vi "path steer61.vi"(11 "lane":bool) -> (2 "curve vel limit":dbl=14.843332236967187, 3 "handle":dbl=-359.09688121459806)   [LabVIEW 2015]
uses:
  G_ALL.vi
  <vilib>/Analysis/polynomials.llb/Scalar Polynomial Evaluation (DBL).vi
  <vilib>/Analysis/polynomials.llb/nth Derivative of Polynomial (DBL).vi
  G_LCM.vi
  <vilib>/Analysis/polynomials.llb/1D Polynomial Evaluation (DBL).vi
  <vilib>/Analysis/NI_AALPro.lvlib
  G_SEN.vi
  <vilib>/gmath/NI_Gmath.lvlib
panel:
  in  "speed gain":dbl=1.0 format="%#_13g"
  in  "lpf gain":dbl=0.1 format="%#_13g"
  out "Waveform Chart":dbl(graph)
  in  "index (row)":i32
  out "dist speed":dbl[](array[numeric])=[-6.280629727990325, -5.767652620171672, -5.260811269352596, -4.750405616087261, -4.247626177640517, -3.7442417201726186, -3.234236998487254, -2.733202494381619, -2.2309876435732536, -1.727969770767316, -1.2170174151123292, -0.7112755506690004, -0.2048354308747279, 0.2980698513495696, 0.8052753145152414, 1.3068201262418702, 1.8071308154794987, 2.3105942059932456, 2.816881132611934, 3.321235349091914, 3.8262467144530254, 4.328309326210711, 4.83288013729348, 5.334580351902129, 5.8405154661100145, 6.344513436357381, 6.84671687285963, 7.347037647467956, 7.85260944831298, 8.355677730085302, 8.85924459600933, 9.36378646133383, 9.871392236798886, 10.379135157785838, 10.885149114578343, 11.386372469681485, 11.889282638845971, 12.390546046536894, 12.8945305329367, 13.394897794033318, 13.897303578434707, 14.398578387722258, 14.903133677335356, 15.408547950712162, 15.909840311837332, 16.412650077140604, 16.91886527417174, 17.42043178538479, 17.928892627599016, 18.429060187867897, 18.938769393907265, 19.44497971039645, 19.95108288625684, 20.458874628420645, 20.966711680341415, 21.468694651165553, 21.97077515459592, 22.476640025076534, 22.986901398368484, 23.490789085466282, 23.998423060461953, 24.50111144191703, 25.010444092843613]
  out "Polynomial Coefficients 2":dbl[](array[numeric])
  out "R0":dbl
  out "handle 2":dbl=-359.09688121459806
  out "dist":dbl[](array[numeric])=[-6.280629727990325, -5.767652620171672, -5.260811269352596, -4.750405616087261, -4.247626177640517, -3.7442417201726186, -3.234236998487254, -2.733202494381619, -2.2309876435732536, -1.727969770767316, -1.2170174151123292, -0.7112755506690004, -0.2048354308747279, 0.2980698513495696, 0.8052753145152414, 1.3068201262418702, 1.8071308154794987, 2.3105942059932456, 2.816881132611934, 3.321235349091914, 3.8262467144530254, 4.328309326210711, 4.83288013729348, 5.334580351902129, 5.8405154661100145, 6.344513436357381, 6.84671687285963, 7.347037647467956, 7.85260944831298, 8.355677730085302, 8.85924459600933, 9.36378646133383, 9.871392236798886, 10.379135157785838, 10.885149114578343, 11.386372469681485, 11.889282638845971, 12.390546046536894, 12.8945305329367, 13.394897794033318, 13.897303578434707, 14.398578387722258, 14.903133677335356, 15.408547950712162, 15.909840311837332, 16.412650077140604, 16.91886527417174, 17.42043178538479, 17.928892627599016, 18.429060187867897, 18.938769393907265, 19.44497971039645, 19.95108288625684, 20.458874628420645, 20.966711680341415, 21.468694651165553, 21.97077515459592, 22.476640025076534, 22.986901398368484, 23.490789085466282, 23.998423060461953, 24.50111144191703, 25.010444092843613]
  in  "ap[g]":dbl=0.01 format="%#_13g"
  in  "mu":dbl=0.35 format="%#_13g"
  in  "an[g]":dbl=-0.03 format="%#_13g"
  out "Waveform Graph 2":dynamicdata(graph)=[{"t0"=timestamp(3558070004.848593 s since 1904-01-01), "dt"=1.0, "Y"=[2.6999392249698047, 1.6951051020445074, 1.0707905056587288, 0.8180527212240709, 0.9190152508675626, 1.2963877361766827, 1.970624056488019, 3.4965104940836413, 201.6, 201.6, 201.6, 201.6, 201.6, 201.6, 201.6, 201.6, 201.6, 201.6, 201.6, 201.6, 201.6, 201.6, 201.6, 201.6, 201.6, 9.532169956190149, 6.2694973959061215, 4.816384979354145, 3.8625477434998605, 3.1463412301935363, 2.568397389060611, 2.09391085834571, 1.7118919309961866, 1.427834339946269, 1.2511128718613436, 1.190295122332855, 1.2494808598163556, 1.4335700986818793, 1.7728772048959551, 2.418642872855935, 5.241778140587992, 201.6, 201.6, 201.6, 201.6, 201.6, 201.6, 201.6, 201.6, 201.6, 201.6, 201.6, 201.6, 201.6, 201.6, 201.6, 201.6, 201.6, 201.6, 201.6, 201.6, 201.6, 201.6]}, {"t0"=timestamp(3558070004.848593 s since 1904-01-01), "dt"=1.0, "Y"=[2.6999392249698047, 1.6951051020445074, 1.0707905056587288, 0.8180527212240709, 0.9190152508675626, 1.2963877361766827, 1.970624056488019, 3.4965104940836413, 20.777549661712815, 20.247536270100138, 19.694565186792815, 19.13150029565853, 18.550539773696645, 17.955042408424784, 17.333744168195455, 16.696661871332914, 16.035950098109442, 15.342378965317303, 14.611756797060403, 13.845642849689991, 13.03348797188081, 12.172479477913956, 11.240920032490967, 10.230903985827208, 9.099530123436892, 7.81122506851608, 6.2694973959061215, 4.816384979354145, 3.8625477434998605, 3.1463412301935363, 2.568397389060611, 2.09391085834571, 1.7118919309961866, 1.427834339946269, 1.2511128718613436, 1.190295122332855, 1.2494808598163556, 1.4335700986818793, 1.7728772048959551, 2.418642872855935, 5.241778140587992, 201.6, 201.6, 201.6, 201.6, 201.6, 201.6, 201.6, 201.6, 201.6, 201.6, 201.6, 201.6, 201.6, 201.6, 201.6, 201.6, 201.6, 201.6, 201.6, 201.6, 201.6, 201.6]}, {"t0"=timestamp(0 s since 1904-01-01), "dt"=1.0, "Y"=[2.6999392249698047, 1.6951051020445074, 1.0707905056587288, 0.8180527212240709, 0.9190152508675626, 1.2963877361766827, 1.970624056488019, 3.4965104940836413, 7.108855050211476, 9.429067355168725, 11.308583683012714, 12.902067626338482, 14.32116957022803, 15.603166352532973, 16.797313219711075, 16.696661871332914, 16.035950098109442, 15.342378965317303, 14.611756797060403, 13.845642849689991, 13.03348797188081, 12.172479477913956, 11.240920032490967, 10.230903985827208, 9.099530123436892, 7.81122506851608, 6.2694973959061215, 4.816384979354145, 3.8625477434998605, 3.1463412301935363, 2.568397389060611, 2.09391085834571, 1.7118919309961866, 1.427834339946269, 1.2511128718613436, 1.190295122332855, 1.2494808598163556, 1.4335700986818793, 1.7728772048959551, 2.418642872855935, 5.241778140587992, 8.106464321213798, 10.208013173205686, 11.948130714804863, 13.453538277833673, 14.81058095698709, 16.061404030280418, 17.21131827924602, 18.303446987203408, 19.317614592377343, 20.299067875936583, 21.228923087902636, 22.11953935666036, 22.978461118838254, 23.806486212234905, 24.597587927766437, 25.364173907146245, 26.113789179785613, 26.848724907341754, 27.555251257689754, 28.249167970580274, 28.919921293974994, 29.58403363562809]}]
  out "map_track for speed":dbl[][](array[numeric])=[[-0.3545450857664302, -6.2388566107065655], [-0.27704582904833586, -5.731767488012998], [-0.20533240909466363, -5.230025183339917], [-0.13399376942622507, -4.724629566643976], [-0.06871872109144915, -4.226105412976658], [-0.005201324439524461, -3.7267443688985153], [0.05648658324735591, -3.2204841411632317], [0.11292137912439827, -2.7226380925511173], [0.1614318645585973, -2.2227716212056117], [0.20611921619876952, -1.7217426590032276], [0.2514800464586248, -1.2128077861289897], [0.2966935930855752, -0.7090910317401496], [0.3370616547081277, -0.204262333528494], [0.37465481783960886, 0.29723589874642653], [0.4044573002719885, 0.803565034690598], [0.43241637259429494, 1.3043299380582118], [0.4571121863051213, 1.8040307510959646], [0.45201550718714745, 2.307468343503967], [0.3863546760099802, 2.809479406443939], [0.25417130196906557, 3.2962038986449116], [0.06111432793630125, 3.7628573931364953], [-0.19013433422201217, 4.19753080604394], [-0.49758286654376527, 4.597614676463535], [-0.8530000954510649, 4.951707459126808], [-1.2554532803579177, 5.2583045461104865], [-1.6928943683564668, 5.508622840575976], [-2.155745510638023, 5.703500011438359], [-2.634513106918592, 5.848766890858279], [-3.129308121801891, 5.952597228699951], [-3.627772088541141, 6.020504297462557], [-4.130029041586696, 6.056802252968919], [-4.634539834160694, 6.06240172093335], [-5.142102959732917, 6.055821687131267], [-5.649843095559644, 6.057503437117642], [-6.155823778443234, 6.063306282752706], [-6.656719729677723, 6.081419751160103], [-7.158588084773581, 6.113773922489787], [-7.651740703683538, 6.203582042123632], [-8.131423336348554, 6.35819424879321], [-8.583409716824091, 6.572846776944994], [-9.005194999840848, 6.845809681440183], [-9.386776083797882, 7.170882459126112], [-9.72476913428849, 7.54549791275371], [-10.011412061388244, 7.961766359884512], [-10.239416063440592, 8.40820583660063], [-10.40783468222519, 8.881970365592638], [-10.516838106738941, 9.376310409640807], [-10.590206702194822, 9.872481765496081], [-10.62912705284488, 10.379450831978916], [-10.637432741269066, 10.879549426143232], [-10.61938203200132, 11.388938910345853], [-10.592347246602534, 11.894426798329851], [-10.558291863385081, 12.399382890965526], [-10.517428444424214, 12.90552776587841], [-10.478548864380736, 13.41187433647924], [-10.440437467355913, 13.912408475588894], [-10.405933723810719, 14.413302000807835], [-10.372241554466061, 14.918043622740504], [-10.343427469450347, 15.427490791324738], [-10.315674147163909, 15.930613593740642], [-10.290940898551378, 16.43764467659748], [-10.26753174415437, 16.939787704369788], [-10.243318891221465, 17.44854450978152]]
  out "Polynomial Coefficients":dbl[](array[numeric])=[0.3514314245197786, 0.08317550338697662, -0.0038021171840465, -0.00346461088477799, -0.0012982677212205788, -0.00011561582792426496]
  out "XY Graph":cluster{"Y":dbl[], "Y":dbl[]}[](graph)=[{"Y"=[-0.3545450857664302, -0.27704582904833586, -0.20533240909466363, -0.13399376942622507, -0.06871872109144915, -0.005201324439524461, 0.05648658324735591, 0.11292137912439827, 0.1614318645585973, 0.20611921619876952, 0.2514800464586248, 0.2966935930855752, 0.3370616547081277, 0.37465481783960886, 0.4044573002719885, 0.43241637259429494, 0.4571121863051213, 0.45201550718714745, 0.3863546760099802, 0.25417130196906557, 0.06111432793630125, -0.19013433422201217, -0.49758286654376527, -0.8530000954510649, -1.2554532803579177, -1.6928943683564668], "Y"=[-6.2388566107065655, -5.731767488012998, -5.230025183339917, -4.724629566643976, -4.226105412976658, -3.7267443688985153, -3.2204841411632317, -2.7226380925511173, -2.2227716212056117, -1.7217426590032276, -1.2128077861289897, -0.7090910317401496, -0.204262333528494, 0.29723589874642653, 0.803565034690598, 1.3043299380582118, 1.8040307510959646, 2.307468343503967, 2.809479406443939, 3.2962038986449116, 3.7628573931364953, 4.19753080604394, 4.597614676463535, 4.951707459126808, 5.2583045461104865, 5.508622840575976]}, {"Y"=[-0.34824861454222367, -0.2838190821086385, -0.21088307053199773, -0.13573975147394757, -0.06474548918773154, 0.0006618412479036939, 0.06025418227747581, 0.11267247761975072, 0.16039640436065217, 0.20497730506502992, 0.2486380781866307, 0.29146844512109193, 0.33431047405158726, 0.3757168715400785, 0.41343550897313974, 0.4415691081325965, 0.4528064519658091, 0.43617827243140883, 0.3771483424612058, 0.2619623140505302, 0.07848992524601944, -0.17634937336605716, -0.5008339909423127, -0.875287479505389, -1.27737354646982, -1.6668168609056053], "Y"=[-6.2388566107065655, -5.731767488012998, -5.230025183339917, -4.724629566643976, -4.226105412976658, -3.7267443688985153, -3.2204841411632317, -2.7226380925511173, -2.2227716212056117, -1.7217426590032276, -1.2128077861289897, -0.7090910317401496, -0.204262333528494, 0.29723589874642653, 0.803565034690598, 1.3043299380582118, 1.8040307510959646, 2.307468343503967, 2.809479406443939, 3.2962038986449116, 3.7628573931364953, 4.19753080604394, 4.597614676463535, 4.951707459126808, 5.2583045461104865, 5.508622840575976]}]
  out "ref":dbl[](array[numeric])=[-29.50710129286377, 0.08298448837840622, 0.3514314245197786]
  in  "gain":dbl[](array[numeric])=[0.7, 1400.0, 750.0]
  out "path end":bool
  out "map_track for steering":dbl[][](array[numeric])=[[-0.3545450857664302, -6.2388566107065655], [-0.27704582904833586, -5.731767488012998], [-0.20533240909466363, -5.230025183339917], [-0.13399376942622507, -4.724629566643976], [-0.06871872109144915, -4.226105412976658], [-0.005201324439524461, -3.7267443688985153], [0.05648658324735591, -3.2204841411632317], [0.11292137912439827, -2.7226380925511173], [0.1614318645585973, -2.2227716212056117], [0.20611921619876952, -1.7217426590032276], [0.2514800464586248, -1.2128077861289897], [0.2966935930855752, -0.7090910317401496], [0.3370616547081277, -0.204262333528494], [0.37465481783960886, 0.29723589874642653], [0.4044573002719885, 0.803565034690598], [0.43241637259429494, 1.3043299380582118], [0.4571121863051213, 1.8040307510959646], [0.45201550718714745, 2.307468343503967], [0.3863546760099802, 2.809479406443939], [0.25417130196906557, 3.2962038986449116], [0.06111432793630125, 3.7628573931364953], [-0.19013433422201217, 4.19753080604394], [-0.49758286654376527, 4.597614676463535], [-0.8530000954510649, 4.951707459126808], [-1.2554532803579177, 5.2583045461104865], [-1.6928943683564668, 5.508622840575976]]
  in  "control point":dbl=0.3 format="%#_13g"
  out "R_new":dbl=-132.87270287440214
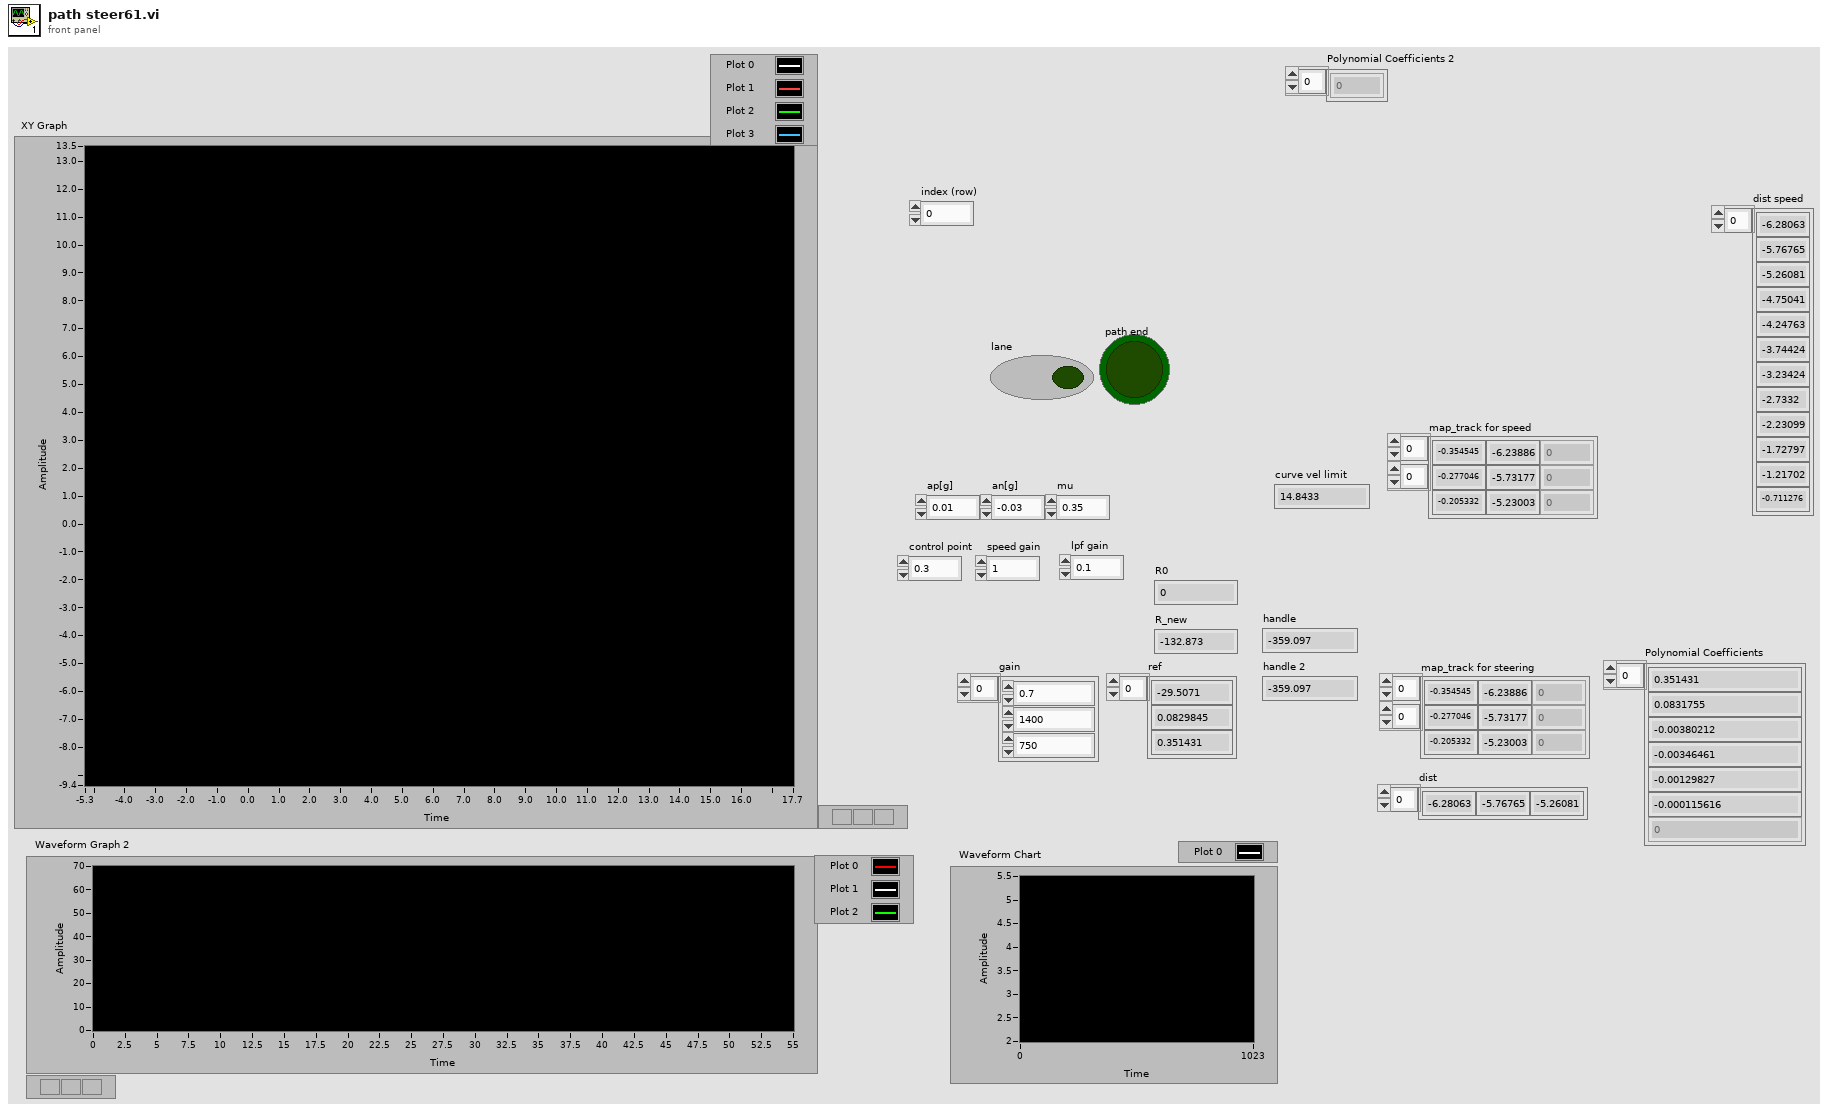
[diagram p1: front panel]
types:
  T1 = cluster{"Steer_input":dbl, "Steer_output":dbl, "VS_des":dbl, "VS_can":dbl, "heading":dbl, "auto":bool, "run":bool, "x":dbl, "y":dbl, "slam_y":dbl, "slam_x":dbl, "slam_heading":dbl}
  T2 = cluster{"C_Wheel base":dbl, "ratio_steer":dbl, "Overall width":dbl, "af":dbl, "turn radius":dbl, "eval":dbl, "ap":dbl, "an":dbl, "Vmax":dbl, "mu":dbl, "Vlast":dbl}
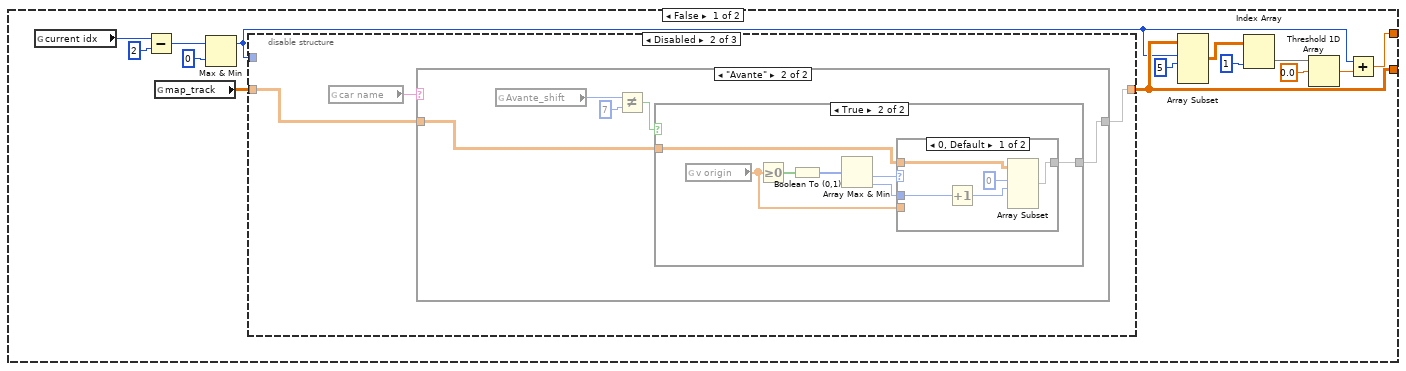
[diagram p2: hidden frame]
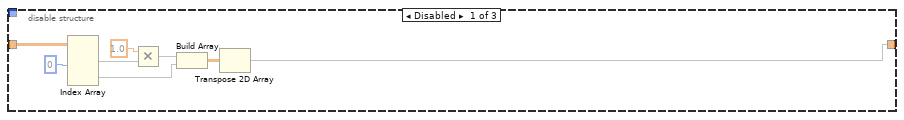
[diagram p3: hidden frame]
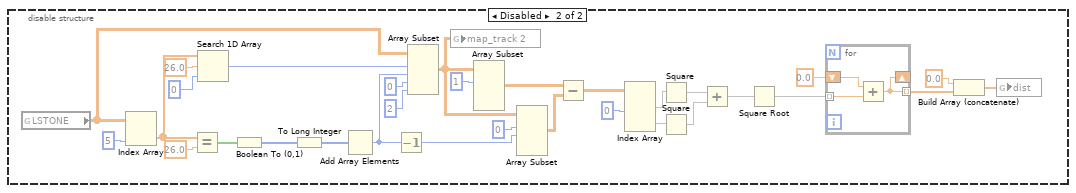
[diagram p8: hidden frame]
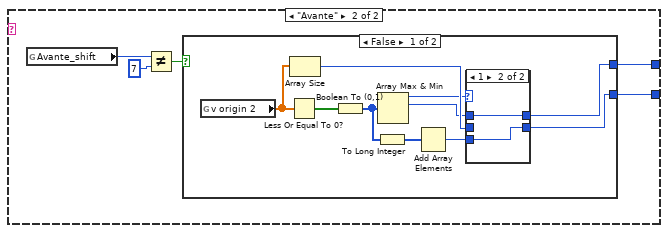
[diagram p11: hidden frame]
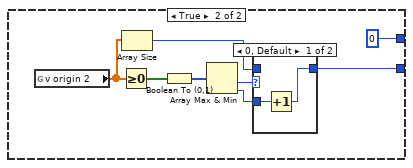
[diagram p13: hidden frame]
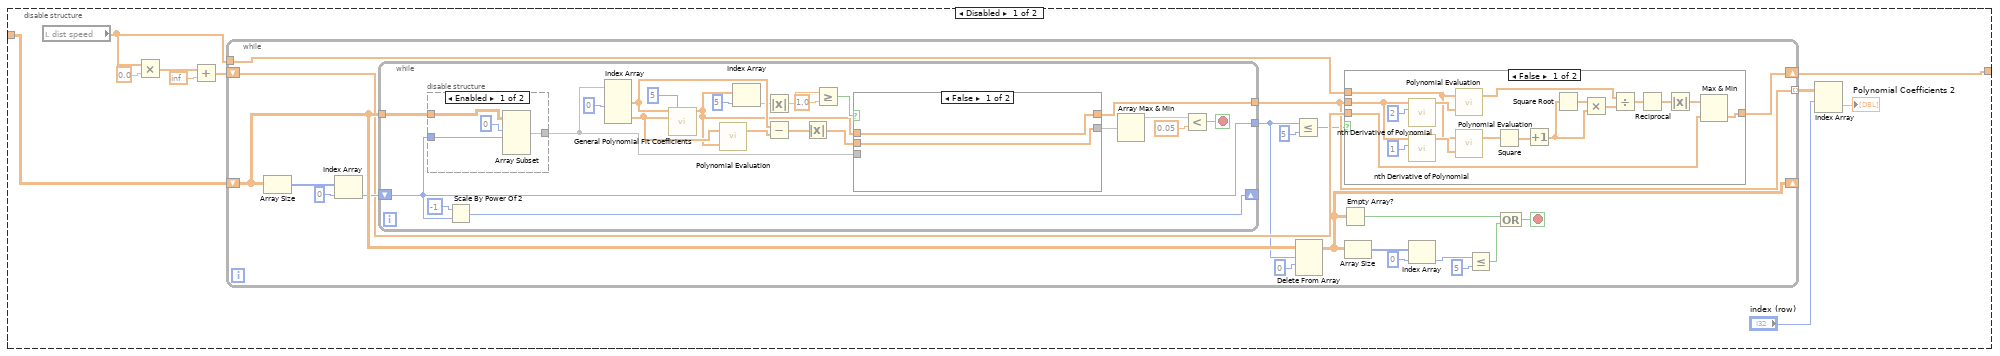
[diagram p15: hidden frame]
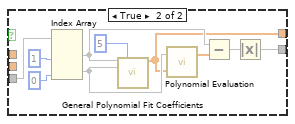
[diagram p17: hidden frame]
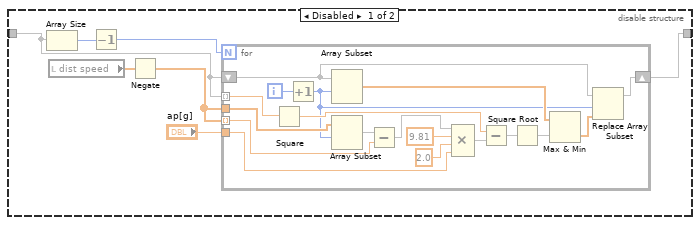
[diagram p19: hidden frame]
diagram:
  n1 = flat-sequence {
    tunnel: [w225] -> w1
    tunnel: w1 -> [w359]
    tunnel: [w437] -> w5
    tunnel: w5 -> [w447]
    tunnel: [w447] -> w4
    tunnel: [w438] -> w3
    tunnel: [w442] -> w2
    tunnel: w4 -> [w480]
    tunnel: w3 -> [w478]
    tunnel: w2 -> [w457]
    frame #0 {
      n2 = disable-structure shown="Enabled" {
        frame Enabled {
          n3 = case shown="True" "lane" {
            tunnel: [w93 w136] -> w31
            tunnel: [w95 _] -> w64
            frame False {
              n4 = global read "G_ALL.vi" "current idx"() -> (w96:i32)
              n5 = Subtract(x=w96, y=2) -> (x-y=w103:i32)
              n6 = global read "G_ALL.vi" "map_track"() -> (w94:dbl[][])
              n7 = Max & Min(x=w103, y=0) -> (max(x,y)=w91:i32)  [unwired: 1 out]
              n8 = disable-structure shown="Disabled" {
                disable-tunnel: w94 -> [w112 w114 w135]
                disable-tunnel: [w105 w113 w135] -> w93
                disable-tunnel: w91 -> [_ _ _]
                frame Disabled {
                  n9 = Index Array(array=w112, index (col) #1=0 ("disabled index (col)")) -> (element #1=w110:dbl[], element #2=w107:dbl[])  [unwired: 3 in]
                  n10 = Multiply(x=1.0, y=w110) -> (x*y=w108:dbl[])
                  n11 = Build Array(w108, w107) -> (w106:dbl[][])
                  n12 = Transpose 2D Array(2D array=w106) -> (transposed array=w105:dbl[][])
                }
                frame Disabled {
                  n13 = global read "G_LCM.vi" "car name"() -> (w115:string)
                  n14 = case shown="\"Avante\"" w115 {
                    tunnel: [w116 w118] -> w113
                    tunnel: w114 -> [w116 w117]
                    frame Default {
                    }
                    frame "Avante" {
                      n15 = global read "G_ALL.vi" "Avante_shift"() -> (w120:u8)
                      n16 = Not Equal?(x=w120, y=u8 7) -> (x != y?=w119:bool)
                      n17 = case shown="True" w119 {
                        tunnel: [_ w124] -> w118
                        tunnel: w117 -> [_ w123]
                        frame False {
                        }
                        frame True {
                          n18 = global read "G_ALL.vi" "v origin"() -> (w125:dbl[])
                          n19 = Greater Or Equal To 0?(x=w125) -> (x >= 0?=w128:bool[])
                          n20 = Boolean To (0,1)(Boolean=w128) -> (0, 1=w127:i16[])
                          n21 = Array Max & Min(array=w127) -> (min value=w126:i16, min index (indices)=w122:i32)  [unwired: 2 out]
                          n22 = case shown="0, Default" w126 {
                            tunnel: w125 -> [_ _]
                            tunnel: [w130 w134] -> w124
                            tunnel: w123 -> [w132 w134]
                            tunnel: w122 -> [w133 _]
                            frame 0, Default {
                              n23 = Increment(x=w133) -> (x+1=w131:i32)
                              n24 = Array Subset(array=w132, index (row)=0 ("index"), length (row)=w131) -> (w130:dbl[][])  [unwired: 2 in]
                            }
                            frame 1 {
                            }
                          }
                        }
                      }
                    }
                  }
                }
                frame Enabled {
                }
              }
              n25 = Array Subset(array=w93, index (row)=w91, length (row)=5 ("length")) -> (w100:dbl[][])  [unwired: 2 in]
              n26 = Index Array(array=w100, index (col)=1 ("disabled index (col)")) -> (element=w98:dbl[])  [unwired: 1 in]
              n27 = Threshold 1D Array(2:0.0 ("threshold y"), 3:w98) -> (0:w92:dbl)  [unwired: 1 in]
              n28 = Add(x=w91, y=w92) -> (x+y=w95:dbl)
            }
            frame True {
              n29 = global read "G_ALL.vi" "map_track lane"() -> (w136:dbl[][])
            }
          }
          n30 = Round Toward -Infinity(1:w64) -> (0:w60:dbl)
          n31 = Index Array(array=w31, index (col) #1=0 ("disabled index (col)")) -> (element #1=w23:dbl[], element #2=w24:dbl[])  [unwired: 3 in]
          n32 = Equal?(x=w60, y=w64) -> (x = y?=w61:bool)
          n33 = To Long Integer(number=w60) -> (32bit integer=w62:i32)
          n34 = Interpolate 1D Array(1:w64, 2:w23) -> (0:w25:dbl)
          n35 = Interpolate 1D Array(1:w64, 2:w24) -> (0:w26:dbl)
          n36 = Increment(x=w62) -> (x+1=w63:i32)
          n37 = Round Toward +Infinity(x=w64) -> (ceil(x): smallest int >= x=w59:dbl)
          n38 = Select(t=w62, s=w61, f=w63) -> (s? t:f=w19:i32)
          n39 = global read "G_ALL.vi" "CARDATA"() -> (w29:T1)
          n40 = Array Subset(array=w31, index (row)=0 ("index"), length (row)=w19) -> (w33:dbl[][])  [unwired: 2 in]
          n41 = Unbundle By Name(w29) -> ("VS_can"=w65:dbl)
          n42 = Index Array(array=w33, index (col) #1=0 ("disabled index (col)")) -> (element #1=w35:dbl[], element #2=w36:dbl[])  [unwired: 3 in]
          n43 = Reverse 1D Array(array=w35) -> (reversed array=w37:dbl[])
          n44 = Reverse 1D Array(array=w36) -> (reversed array=w38:dbl[])
          n45 = Multiply(x=2.0, y=w65) -> (x*y=w66:dbl)
          n46 = Build Array(w37, w38) -> (w57:dbl[][])
          n47 = To Long Integer(number=w59) -> (32bit integer=w10:i32)
          n48 = Max & Min(x=w66, y=25.0) -> (max(x,y)=w30:dbl)  [unwired: 1 out]
          n49 = Array Subset(array=w31, index (row)=w10) -> (w55:dbl[][])  [unwired: 3 in]
          n50 = Transpose 2D Array(2D array=w57) -> (transposed array=w58:dbl[][])
          n51 = Build Array(w25, w26) -> (w40:dbl[])
          n52 = for {
            tunnel: w58 -> [w73] mode=indexing
            shift-right: [w73] -> _
            shift-left: w40 -> [w80]
            shift-right: [w72] -> _
            shift-left: 0.0 -> [w75]
            tunnel: 15.0 ("y") -> [w74]
            tunnel: [w72] -> w44 mode=indexing
            stop <- w71 stop-if-true
            n53 = Subtract(x=w73, y=w80) -> (x-y=w79:dbl[])
            n54 = Square(x=w79) -> (x^2=w78:dbl[])
            n55 = Add Array Elements(numeric array=w78) -> (sum=w77:dbl)
            n56 = Square Root(x=w77) -> (sqrt(x)=w76:dbl)
            n57 = Add(x=w75, y=w76) -> (x+y=w72:dbl)
            n58 = Greater Or Equal?(x=w72, y=w74) -> (x >= y?=w71:bool)
          }
          n59 = for {
            tunnel: w55 -> [w83] mode=indexing
            shift-right: [w83] -> _
            shift-left: w40 -> [w90]
            shift-right: [w82] -> _
            shift-left: 0.0 -> [w85]
            tunnel: w30 -> [w84]
            tunnel: [w82] -> w56 mode=indexing
            tunnel: [w81] -> w69
            stop <- w81 stop-if-true
            n60 = Subtract(x=w83, y=w90) -> (x-y=w89:dbl[])
            n61 = Square(x=w89) -> (x^2=w88:dbl[])
            n62 = Add Array Elements(numeric array=w88) -> (sum=w87:dbl)
            n63 = Square Root(x=w87) -> (sqrt(x)=w86:dbl)
            n64 = Add(x=w85, y=w86) -> (x+y=w82:dbl)
            n65 = Greater Or Equal?(x=w82, y=w84) -> (x >= y?=w81:bool)
          }
          n66 = global read "G_ALL.vi" "v origin"() -> (w11:dbl[])
          n67 = Array Subset(array=w11, index=0, length=w19) -> (w17:dbl[])
          n68 = Negate(x=w44) -> (-x=w42:dbl[])
          n69 = Not(x=w69) -> (.not. x?=→"path end":bool)
          n70 = Array Size(array=w44) -> (size(s)=w14:i32)
          n71 = Array Size(array=w56) -> (size(s)=w9:i32)
          n72 = Reverse 1D Array(array=w17) -> (reversed array=w16:dbl[])
          n73 = Array Subset(array=w11, index=w10, length=w9) -> (w8:dbl[])
          n74 = Reverse 1D Array(array=w42) -> (reversed array=w43:dbl[])
          n75 = Array Subset(array=w58, index (row)=0 ("index"), length (row)=w14) -> (w50:dbl[][])  [unwired: 2 in]
          n76 = Array Subset(array=w55, index (row)=0 ("index"), length (row)=w9) -> (w68:dbl[][])  [unwired: 2 in]
          n77 = Build Array (concatenate)(w43, w56) -> (w20:dbl[])
          n78 = Array Subset(array=w16, index=0, length=w14) -> (w13:dbl[])
          n79 = global write "G_ALL.vi" "dist"(w20) -> ()
          n80 = Reverse 1D Array(array=w13) -> (reversed array=w12:dbl[])
          n81 = Index Array(array=w50, index (col) #1=0 ("disabled index (col)")) -> (element #1=w51:dbl[], element #2=w52:dbl[])  [unwired: 3 in]
          n82 = Reverse 1D Array(array=w51) -> (reversed array=w48:dbl[])
          n83 = Reverse 1D Array(array=w52) -> (reversed array=w47:dbl[])
          n84 = Build Array (concatenate)(w12, w8) -> (w7:dbl[])
          n85 = Build Array(w48, w47) -> (w46:dbl[][])
          n86 = global write "G_ALL.vi" "v origin 2"(w7) -> ()
          n87 = Transpose 2D Array(2D array=w46) -> (transposed array=w53:dbl[][])
          n88 = Build Array (concatenate)(w53, w68) -> (w21:dbl[][])
          n89 = global write "G_ALL.vi" "map_track 2"(w21) -> ()
        }
        frame Disabled {
          n90 = global read "G_SEN.vi" "LSTONE"() -> (w159:sgl[][])
          n91 = Index Array(array=w159, index (col)=5 ("disabled index (col)")) -> (element=w165:sgl[])  [unwired: 1 in]
          n92 = Equal?(x=w165, y=sgl 26.0 ("element")) -> (x = y?=w163:bool[])
          n93 = Search 1D Array(1D array=w165, element=sgl 26.0, start index (0)=0) -> (index of element=w158:i32)
          n94 = Boolean To (0,1)(Boolean=w163) -> (0, 1=w161:i16[])
          n95 = To Long Integer(number=w161) -> (32bit integer=w160:i32[])
          n96 = Add Array Elements(numeric array=w160) -> (sum=w153:i32)
          n97 = Decrement(x=w153) -> (x-1=w152:i32)
          n98 = Array Subset(array=w159, index (row)=w158, length (row)=w153, index (col)=0 ("index"), length (col)=2 ("length")) -> (w154:sgl[][])
          n99 = global write "G_ALL.vi" "map_track 2"(w154) -> ()
          n100 = Array Subset(array=w154, index (row)=1 ("index")) -> (w149:sgl[][])  [unwired: 3 in]
          n101 = Array Subset(array=w154, index (row)=0 ("index"), length (row)=w152) -> (w150:sgl[][])  [unwired: 2 in]
          n102 = Subtract(x=w149, y=w150) -> (x-y=w148:sgl[][])
          n103 = Index Array(array=w148, index (col) #1=0 ("disabled index (col)")) -> (element #1=w146:sgl[], element #2=w145:sgl[])  [unwired: 3 in]
          n104 = Square(x=w146) -> (x^2=w143:sgl[])
          n105 = Square(x=w145) -> (x^2=w144:sgl[])
          n106 = Add(x=w143, y=w144) -> (x+y=w142:sgl[])
          n107 = Square Root(x=w142) -> (sqrt(x)=w141:sgl[])
          n108 = for {
            tunnel: w141 -> [w170] mode=indexing
            shift-right: [w168] -> _
            shift-left: sgl 0.0 -> [w169]
            tunnel: [w168] -> w139 mode=indexing
            n109 = Add(x=w169, y=w170) -> (x+y=w168:sgl)
          }
          n110 = Build Array (concatenate)(sgl 0.0, w139) -> (w137:sgl[])
          n111 = global write "G_ALL.vi" "dist"(w137) -> ()
        }
      }
    }
    frame #1 {
      n112 = disable-structure shown="Disabled" {
        disable-tunnel: [w193 _] -> w182
        frame Disabled {
          n113 = global read "G_LCM.vi" "car name"() -> (w193:string)
        }
        frame Enabled {
        }
      }
      n114 = case shown="\"False\", Default" w182 {
        tunnel: [w194 w198] -> w178
        tunnel: [_ w197] -> w177
        frame "False", Default {
          n115 = global read "G_ALL.vi" "dist"() -> (w195:dbl[])
          n116 = Array Size(array=w195) -> (size(s)=w194:i32)
        }
        frame "Avante" {
          n117 = global read "G_ALL.vi" "Avante_shift"() -> (w199:u8)
          n118 = Not Equal?(x=w199, y=u8 7) -> (x != y?=w196:bool)
          n119 = case shown="False" w196 {
            tunnel: [w204 w219] -> w198
            tunnel: [w208 0] -> w197
            frame False {
              n120 = global read "G_ALL.vi" "v origin 2"() -> (w210:dbl[])
              n121 = Less Or Equal To 0?(x=w210) -> (x <= 0?=w205:bool[])
              n122 = Array Size(array=w210) -> (size(s)=w209:i32)
              n123 = Boolean To (0,1)(Boolean=w205) -> (0, 1=w202:i16[])
              n124 = To Long Integer(number=w202) -> (32bit integer=w201:i32[])
              n125 = Array Max & Min(array=w202) -> (max value=w206:i16, max index (indices)=w207:i32)  [unwired: 2 out]
              n126 = Add Array Elements(numeric array=w201) -> (sum=w203:i32)
              n127 = case shown="1" w206 {
                tunnel: w209 -> [w211 _]
                tunnel: [_ w213] -> w208
                tunnel: w207 -> [_ w213]
                tunnel: [w211 w212] -> w204
                tunnel: w203 -> [_ w212]
                frame 0, Default {
                }
                frame 1 {
                }
              }
            }
            frame True {
              n128 = global read "G_ALL.vi" "v origin 2"() -> (w216:dbl[])
              n129 = Greater Or Equal To 0?(x=w216) -> (x >= 0?=w221:bool[])
              n130 = Array Size(array=w216) -> (size(s)=w220:i32)
              n131 = Boolean To (0,1)(Boolean=w221) -> (0, 1=w218:i16[])
              n132 = Array Max & Min(array=w218) -> (min value=w217:i16, min index (indices)=w214:i32)  [unwired: 2 out]
              n133 = case shown="0, Default" w217 {
                tunnel: w220 -> [_ w224]
                tunnel: [w223 w224] -> w219
                tunnel: w214 -> [w222 _]
                frame 0, Default {
                  n134 = Increment(x=w222) -> (x+1=w223:i32)
                }
                frame 1 {
                }
              }
            }
          }
        }
      }
      n135 = global read "G_ALL.vi" "dist"() -> (w181:dbl[])
      n136 = Array Subset(array=w181, index=w177, length=w178) -> (w173:dbl[])
      n137 = Threshold 1D Array(2:-3.0 ("threshold y"), 3:w173) -> (0:w190:dbl)  [unwired: 1 in]
      n138 = Round Toward -Infinity(1:w190) -> (0:w191:dbl)
      n139 = To Long Integer(number=w191) -> (32bit integer=w171:i32)
      n140 = Array Subset(array=w173, index=w171) -> (→"dist speed":dbl[])  [unwired: 1 in]
      n141 = global read "G_ALL.vi" "map_track 2"() -> (w180:dbl[][])
      n142 = Threshold 1D Array(1:w171, 2:6.0 ("threshold y"), 3:w173) -> (0:w186:dbl)
      n143 = Round Toward +Infinity(x=w186) -> (ceil(x): smallest int >= x=w185:dbl)
      n144 = To Long Integer(number=w185) -> (32bit integer=w187:i32)
      n145 = Array Subset(array=w180, index (row)=w177) -> (w179:dbl[][])  [unwired: 3 in]
      n146 = Subtract(x=w187, y=w171) -> (x-y=w188:i32)
      n147 = Array Subset(array=w179, index (row)=w171) -> (w176:dbl[][])  [unwired: 3 in]
      n148 = Increment(x=w188) -> (x+1=w174:i32)
      n149 = disable-structure shown="Enabled" {
        disable-tunnel: w176 -> [w192 _]
        frame Enabled {
          "map_track for speed" <- w192
        }
        frame Disabled {
        }
      }
      n150 = Array Subset(array=w173, index=w171, length=w174) -> (→"dist":dbl[])
      n151 = Array Subset(array=w179, index (row)=w171, length (row)=w174) -> (→"map_track for steering":dbl[][])  [unwired: 2 in]
    }
    frame #2 {
      n152 = local read "map_track for speed"() -> (w226:dbl[][])
      n153 = disable-structure shown="Enabled" {
        disable-tunnel: w226 -> [w236 w315]
        disable-tunnel: [w230 w316] -> w225
        frame Disabled {
          n154 = local read "dist speed"() -> (w235:dbl[])
          n155 = Multiply(x=w235, y=0.0) -> (x*y=w233:dbl[])
          n156 = Add(x=w233, y=inf) -> (x+y=w231:dbl[])
          n157 = while {
            shift-right: [w247] -> _
            shift-left: w236 -> [w254]
            tunnel: w235 -> [w251]
            shift-right: [w248] -> w230
            shift-left: w231 -> [w250]
            tunnel: [w249] -> w229 mode=indexing
            stop <- w241 stop-if-true
            n158 = Array Size(array=w254) -> (size(s)=w256:i32[])
            n159 = Index Array(array=w256, index=0) -> (element=w252:i32)
            n160 = while {
              tunnel: w254 -> [w291]
              shift-right: [w289] -> _
              shift-left: w252 -> [w285]
              tunnel: [w285] -> w237
              tunnel: [w278] -> w249
              stop <- w287 stop-if-true
              n161 = disable-structure shown="Enabled" {
                disable-tunnel: w291 -> [w312 w314]
                disable-tunnel: [w311 w314] -> w284
                disable-tunnel: w285 -> [w310 _]
                frame Enabled {
                  n162 = Array Subset(array=w312, index (row)=0 ("index"), length (row)=w310) -> (w311:dbl[][])  [unwired: 2 in]
                }
                frame Disabled {
                }
              }
              n163 = Scale By Power Of 2(n=i16 -1, x=w285) -> (x*2^n=w289:i32)
              n164 = Index Array(array=w284, index (col) #1=0 ("disabled index (col)")) -> (element #1=w295:dbl[], element #2=w293:dbl[])  [unwired: 3 in]
              n165 = call <vilib>:"General Polynomial Fit Coefficients.vi"("Y"=w295, "polynomial order"=5, "X"=w293) -> ("Polynomial Coefficients"=w277:dbl[])  [unwired: 11 in, 1 out]
              n166 = call-poly <vilib>:"Polynomial Evaluation.vi"("P(x)"=w277, "A"=w293) -> ("P(A)"=w292:dbl[])  [unwired: 1 out]
              n167 = Index Array(array=w277, index=5) -> (element=w276:dbl)
              n168 = Absolute Value(x=w276) -> (abs(x)=w275:dbl)
              n169 = Subtract(x=w295, y=w292) -> (x-y=w294:dbl[])
              n170 = Absolute Value(x=w294) -> (abs(x)=w279:dbl[])
              n171 = Greater Or Equal?(x=w275, y=1.0) -> (x >= y?=w281:bool)
              n172 = case shown="False" w281 {
                tunnel: w284 -> [_ w303]
                tunnel: [w299 w301] -> w280
                tunnel: w279 -> [w299 _]
                tunnel: [w298 w300] -> w278
                tunnel: w277 -> [w298 _]
                frame False {
                }
                frame True {
                  n173 = Index Array(array=w303, index (col) #1=1 ("disabled index (col)"), index (col) #2=0 ("index (col)")) -> (element #1=w306:dbl[], element #2=w308:dbl[])  [unwired: 2 in]
                  n174 = call <vilib>:"General Polynomial Fit Coefficients.vi"("Y"=w306, "polynomial order"=5, "X"=w308) -> ("Polynomial Coefficients"=w300:dbl[])  [unwired: 11 in, 1 out]
                  n175 = call-poly <vilib>:"Polynomial Evaluation.vi"("P(x)"=w300, "A"=w308) -> ("P(A)"=w309:dbl[])  [unwired: 1 out]
                  n176 = Subtract(x=w306, y=w309) -> (x-y=w307:dbl[])
                  n177 = Absolute Value(x=w307) -> (abs(x)=w301:dbl[])
                }
              }
              n178 = Array Max & Min(array=w280) -> (max value=w288:dbl)  [unwired: 3 out]
              n179 = Less?(x=w288, y=0.05) -> (x < y?=w287:bool)
            }
            n180 = Less Or Equal?(x=w237, y=5) -> (x <= y?=w238:bool)
            n181 = Delete From Array(array=w254, length=w237, index (row)=0) -> (array with subset deleted=w247:dbl[][])  [unwired: 1 in, 1 out]
            n182 = Empty Array?(array=w247) -> (empty?=w243:bool)
            n183 = case shown="False" w238 {
              tunnel: w251 -> [w262 _]
              tunnel: w250 -> [w260 w274]
              tunnel: w249 -> [w258 _]
              tunnel: [w257 w274] -> w248
              frame False {
                n184 = call-poly <vilib>:"nth Derivative of Polynomial.vi"("order"=2, "P(x)"=w258) -> ("Nth Derivative of P(x)"=w265:dbl[])  [unwired: 8 in, 1 out]
                n185 = call-poly <vilib>:"nth Derivative of Polynomial.vi"("order"=1, "P(x)"=w258) -> ("Nth Derivative of P(x)"=w267:dbl[])  [unwired: 8 in, 1 out]
                n186 = call-poly <vilib>:"Polynomial Evaluation.vi"("P(x)"=w265, "A"=w262) -> ("P(A)"=w263:dbl[])  [unwired: 1 out]
                n187 = call-poly <vilib>:"Polynomial Evaluation.vi"("P(x)"=w267, "A"=w262) -> ("P(A)"=w271:dbl[])  [unwired: 1 out]
                n188 = Square(x=w271) -> (x^2=w268:dbl[])
                n189 = Increment(x=w268) -> (x+1=w270:dbl[])
                n190 = Square Root(x=w270) -> (sqrt(x)=w269:dbl[])
                n191 = Multiply(x=w269, y=w270) -> (x*y=w266:dbl[])
                n192 = Divide(x=w263, y=w266) -> (x/y=w273:dbl[])
                n193 = Reciprocal(x=w273) -> (1/x=w261:dbl[])
                n194 = Absolute Value(x=w261) -> (abs(x)=w259:dbl[])
                n195 = Max & Min(x=w259, y=w260) -> (min(x,y)=w257:dbl[])  [unwired: 1 out]
              }
              frame True {
              }
            }
            n196 = Array Size(array=w247) -> (size(s)=w246:i32[])
            n197 = Index Array(array=w246, index=0) -> (element=w240:i32)
            n198 = Less Or Equal?(x=w240, y=5) -> (x <= y?=w242:bool)
            n199 = Compound Arithmetic op=OR(w243, w242) -> (w241:bool)
          }
          n200 = Index Array(array=w229, index (row)="index (row)") -> (element=→"Polynomial Coefficients 2":dbl[])  [unwired: 1 in]
        }
        frame Enabled {
          n201 = Array Size(array=w315) -> (size(s)=w323:i32[])
          n202 = Index Array(array=w323, index=0) -> (element=w321:i32)
          n203 = local read "dist speed"() -> (w318:dbl[])
          n204 = Subtract(x=w321, y=2) -> (x-y=w319:i32)
          n205 = for {
            N: w319 -> [_]
            tunnel: w315 -> [w336]
            tunnel: [w328] -> w316 mode=indexing
            tunnel: w318 -> [w327]
            tunnel: [w324] -> w317 mode=indexing
            i -> [w326]
            n206 = Increment(x=w326) -> (x+1=w325:i32)
            n207 = Array Subset(array=w336, index (row)=w326, length (row)=3 ("length")) -> (w334:dbl[][])  [unwired: 2 in]
            n208 = Index Array(array=w327, index=w325) -> (element=w324:dbl)
            n209 = Index Array(array=w334, index (col) #1=0 ("disabled index (col)")) -> (element #1=w332:dbl[], element #2=w331:dbl[])  [unwired: 3 in]
            n210 = Multiply(x=w331, y=0.0) -> (x*y=w330:dbl[])
            n211 = call <vilib>:"Fitting on a Sphere.vi"("Z"=w330, "Y"=w331, "X"=w332) -> ("r"=w328:dbl)  [unwired: 2 out]
          }
          n212 = local write "dist speed"(w317) -> ()
        }
      }
    }
    frame #3 {
      (unwired) 1 ("index")
      n213 = Compound Arithmetic op=MULTIPLY(w359, 9.81 ("value"), "mu") -> (w371:dbl[])
      n214 = Square Root(x=w371) -> (sqrt(x)=w357:dbl[])
      n215 = In Range and Coerce(upper limit=56.0 ("value"), x=w357, lower limit=0.5) -> (coerced(x)=w358:dbl[])  [unwired: 1 out]
      n216 = local read "path end"() -> (w378:bool)
      n217 = call "Convert to Dynamic Data6"("Array"=w358) -> ("Dynamic Data Type"=w362:dynamicdata)  [unwired: 3 in]
      n218 = Reverse 1D Array(array=w358) -> (reversed array=w379:dbl[])
      n219 = case shown="True" w378 {
        tunnel: w379 -> [w407 w411]
        tunnel: [w407 w410] -> w380
        frame False {
        }
        frame True {
          n220 = Replace Array Subset(array=w411, new element=0.0 ("new element/subarray"), index=0) -> (w410:dbl[])
        }
      }
      n221 = local read "dist speed"() -> (w360:dbl[])
      n222 = Array Size(array=w380) -> (size(s)=w376:i32)
      n223 = Reverse 1D Array(array=w360) -> (reversed array=w373:dbl[])
      n224 = Decrement(x=w376) -> (x-1=w375:i32)
      n225 = Negate(x=w373) -> (-x=w374:dbl[])
      n226 = for {
        N: w375 -> [_]
        tunnel: w380 -> [w427] mode=indexing
        tunnel: w374 -> [w428]
        shift-right: [w418] -> w364
        shift-left: w380 -> [w421]
        tunnel: w374 -> [w415] mode=indexing
        tunnel: "an[g]" -> [w412]
        i -> [w429]
        n227 = Square(x=w427) -> (x^2=w426:dbl)
        n228 = Increment(x=w429) -> (x+1=w420:i32)
        n229 = Array Subset(array=w421, index=w420) -> (w422:dbl[])  [unwired: 1 in]
        n230 = Array Subset(array=w428, index=w420) -> (w416:dbl[])  [unwired: 1 in]
        n231 = Subtract(x=w416, y=w415) -> (x-y=w414:dbl[])
        n232 = Compound Arithmetic op=MULTIPLY(w414, 9.81 ("value"), 2.0 ("value"), w412) -> (w424:dbl[])
        n233 = Subtract(x=w426, y=w424) -> (x-y=w423:dbl[])
        n234 = Square Root(x=w423) -> (sqrt(x)=w417:dbl[])
        n235 = Max & Min(x=w422, y=w417) -> (min(x,y)=w419:dbl[])  [unwired: 1 out]
        n236 = Replace Array Subset(array=w421, new element=w419, index=w420) -> (w418:dbl[])
      }
      n237 = Reverse 1D Array(array=w364) -> (reversed array=w350:dbl[])
      n238 = call "Convert to Dynamic Data5"("Array"=w350) -> ("Dynamic Data Type"=w361:dynamicdata)  [unwired: 3 in]
      n239 = disable-structure shown="Enabled" {
        disable-tunnel: [w383 w406] -> w351
        disable-tunnel: w350 -> [w382 w406]
        frame Disabled {
          n240 = Array Size(array=w382) -> (size(s)=w386:i32)
          n241 = local read "dist speed"() -> (w381:dbl[])
          n242 = Decrement(x=w386) -> (x-1=w387:i32)
          n243 = Negate(x=w381) -> (-x=w384:dbl[])
          n244 = for {
            N: w387 -> [_]
            tunnel: w382 -> [w403] mode=indexing
            tunnel: w384 -> [w404]
            shift-right: [w394] -> w383
            shift-left: w382 -> [w397]
            tunnel: w384 -> [w391] mode=indexing
            tunnel: "ap[g]" -> [w388]
            i -> [w405]
            n245 = Square(x=w403) -> (x^2=w402:dbl)
            n246 = Increment(x=w405) -> (x+1=w396:i32)
            n247 = Array Subset(array=w397, index=w396) -> (w398:dbl[])  [unwired: 1 in]
            n248 = Array Subset(array=w404, index=w396) -> (w392:dbl[])  [unwired: 1 in]
            n249 = Subtract(x=w392, y=w391) -> (x-y=w390:dbl[])
            n250 = Compound Arithmetic op=MULTIPLY(w390, 9.81 ("value"), 2.0 ("value"), w388) -> (w400:dbl[])
            n251 = Subtract(x=w402, y=w400) -> (x-y=w399:dbl[])
            n252 = Square Root(x=w399) -> (sqrt(x)=w393:dbl[])
            n253 = Max & Min(x=w398, y=w393) -> (min(x,y)=w395:dbl[])  [unwired: 1 out]
            n254 = Replace Array Subset(array=w397, new element=w395, index=w396) -> (w394:dbl[])
          }
        }
        frame Enabled {
        }
      }
      n255 = local read "control point"() -> (w337:dbl)
      n256 = local read "dist speed"() -> (w352:dbl[])
      n257 = Threshold 1D Array(2:w337, 3:w352) -> (0:w369:dbl)  [unwired: 1 in]
      n258 = call "Convert to Dynamic Data7"("Array"=w351) -> ("Dynamic Data Type"=w365:dynamicdata)  [unwired: 3 in]
      n259 = Interpolate 1D Array(1:w369, 2:w351) -> (0:w339:dbl)
      n260 = Not A Number/Path/Refnum?(number/path/refnum=w339) -> (NaN/Path/Refnum?=w341:bool)
      n261 = Merge Signals(w362, w361, w365) -> (w367:dynamicdata)
      n262 = Select(t=0.0, s=w341, f=w339) -> (s? t:f=w338:dbl)
      n263 = Multiply(x=w367, y=3.6) -> (x*y=→"Waveform Graph 2":dynamicdata)
      n264 = Decrement(x="lpf gain") -> (x-1=w347:dbl)
      n265 = Multiply(x=w338, y=3.6) -> (x*y=w349:dbl)
      n266 = Multiply(x=w349, y="lpf gain") -> (x*y=w345:dbl)
      n267 = feedback #1(0.0) -> (w346:dbl)
      n268 = Multiply(x=w347, y=w346) -> (x*y=w344:dbl)
      n269 = Subtract(x=w345, y=w344) -> (x-y=w342:dbl)
      n270 = feedback-in #1(w342) -> ()
      n271 = Multiply(x=w342, y="speed gain") -> (x*y=→"curve vel limit" →"Waveform Chart":dbl)
    }
    frame #4 {
      n272 = local read "map_track for steering"() -> (w436:dbl[][])
      n273 = Index Array(array=w436, index (col) #1=0 ("disabled index (col)")) -> (element #1=w433:dbl[], element #2=w434:dbl[])  [unwired: 3 in]
      n274 = call <vilib>:"General Polynomial Fit Coefficients.vi"("Y"=w433, "polynomial order"=5, "X"=w434) -> ("Polynomial Coefficients"=w430:dbl[])  [unwired: 11 in, 1 out]
      "Polynomial Coefficients" <- w430
      n275 = call-poly <vilib>:"Polynomial Evaluation.vi"("P(x)"=w430, "a"=0.0) -> ("P(a)"=w437:dbl)  [unwired: 1 out]
    }
    frame #5 {
      n276 = global read "G_LCM.vi" "car name"() -> (w443:string)
      n277 = case shown="\"Avante\"" w443 {
        tunnel: [w448 w451] -> w442
        frame Default {
          n278 = global read "G_ALL.vi" "CARDATA"() -> (w450:T1)
          n279 = Unbundle By Name(w450) -> ("VS_can"=w449:dbl)
          n280 = Less Than 0?(x=w449) -> (x < 0?=w448:bool)
        }
        frame "Avante" {
          n281 = global read "G_ALL.vi" "Avante_shift"() -> (w453:u8)
          n282 = Equal?(x=w453, y=u8 7) -> (x = y?=w451:bool)
        }
      }
      n283 = local read "Polynomial Coefficients"() -> (w446:dbl[])
      n284 = Negate(x="control point") -> (-x=w441:dbl)
      n285 = Select(t=w441, s=w442, f="control point") -> (s? t:f=w439:dbl)
      n286 = call-poly <vilib>:"nth Derivative of Polynomial.vi"("order"=1, "P(x)"=w446) -> ("Nth Derivative of P(x)"=w444:dbl[])  [unwired: 8 in, 1 out]
      n287 = call-poly <vilib>:"Polynomial Evaluation.vi"("P(x)"=w444, "a"=w439) -> ("P(a)"=w438:dbl)  [unwired: 1 out]
    }
    frame #6 {
      n288 = Square(x=w478) -> (x^2=w505:dbl)
      n289 = global read "G_ALL.vi" "CARDATA"() -> (w477:T1)
      n290 = Increment(x=w505) -> (x+1=w503:dbl)
      n291 = local read "Polynomial Coefficients"() -> (w479:dbl[])
      n292 = local read "Polynomial Coefficients"() -> (w463:dbl[])
      n293 = Unbundle By Name(w477) -> ("VS_can"=w476:dbl)
      n294 = Square Root(x=w503) -> (sqrt(x)=w504:dbl)
      n295 = Multiply(x=w504, y=w503) -> (x*y=w502:dbl)
      n296 = local read "control point"() -> (w460:dbl)
      n297 = Divide(x=w476, y=3.6) -> (x/y=w497:dbl)
      n298 = Absolute Value(x=w497) -> (abs(x)=w500:dbl)
      n299 = call-poly <vilib>:"nth Derivative of Polynomial.vi"("order"=2, "P(x)"=w479) -> ("Nth Derivative of P(x)"=w458:dbl[])  [unwired: 8 in, 1 out]
      n300 = Index Array(array=w463, index=1) -> (element=w461:dbl)
      n301 = call-poly <vilib>:"Polynomial Evaluation.vi"("P(x)"=w458, "a"=w460) -> ("P(a)"=w459:dbl)  [unwired: 1 out]
      n302 = Square(x=w461) -> (x^2=w466:dbl)
      n303 = Inverse Tangent(1:w461) -> (0:w456:dbl)
      n304 = Max & Min(x=w500, y=1.0) -> (max(x,y)=w498:dbl)  [unwired: 1 out]
      n305 = global read "G_ALL.vi" "CARSPEC"() -> (w492:T2)
      n306 = Divide(x=w480, y=w498) -> (x/y=w481:dbl)
      n307 = Divide(x=w502, y=w459) -> (x/y=w484:dbl)
      "R_new" <- w484
      n308 = Negate(x=w456) -> (-x=w455:dbl)
      n309 = Increment(x=w466) -> (x+1=w468:dbl)
      n310 = Unbundle By Name(w492) -> ("ratio_steer"=w494:dbl, "C_Wheel base"=w493:dbl)
      n311 = Select(t=w456, s=w457, f=w455) -> (s? t:f=w482:dbl)
      n312 = Square Root(x=w468) -> (sqrt(x)=w467:dbl)
      n313 = Multiply(x=w467, y=w468) -> (x*y=w465:dbl)
      n314 = Divide(x=w493, y=w484) -> (x/y=w486:dbl)
      n315 = Divide(x=w465, y=w459) -> (x/y=→"R0":dbl)
      n316 = Inverse Tangent(1:w486) -> (0:w488:dbl)
      n317 = Multiply(x=180.0 ("y"), y=w488) -> (x*y=w489:dbl)
      n318 = Divide(x=w489, y=3.141592653589793) -> (x/y=w491:dbl)
      n319 = Multiply(x=w494, y=w491) -> (x*y=w485:dbl)
      n320 = Not A Number/Path/Refnum?(number/path/refnum=w485) -> (NaN/Path/Refnum?=w495:bool)
      n321 = Select(t=0.0, s=w495, f=w485) -> (s? t:f=w483:dbl)
      n322 = Build Array(w483, w482, w481) -> (w474:dbl[])
      "ref" <- w474
      n323 = Multiply(x=w474, y="gain") -> (x*y=w454:dbl[])
      n324 = Add Array Elements(numeric array=w454) -> (sum=w473:dbl)
      "handle 2" <- w473
      n325 = Negate(x=w473) -> (-x=w472:dbl)
      n326 = In Range and Coerce(upper limit=479.0, x=w472, lower limit=-479.0) -> (coerced(x)=→"handle":dbl)  [unwired: 1 out]
    }
    frame #7 {
      n327 = local read "dist"() -> (w507:dbl[])
      n328 = local read "map_track for speed"() -> (w521:dbl[][])
      n329 = global write "G_ALL.vi" "Steering dist"(w507) -> ()
      n330 = local read "Polynomial Coefficients"() -> (w510:dbl[])
      n331 = Index Array(array=w521, index (col) #1=0 ("disabled index (col)")) -> (element #1=w519:dbl[], element #2=w511:dbl[])  [unwired: 3 in]
      n332 = local read "R0"() -> (w512:dbl)
      n333 = call-poly <vilib>:"Polynomial Evaluation.vi"("P(x)"=w510, "A"=w511) -> ("P(A)"=w515:dbl[])  [unwired: 1 out]
      n334 = call "Convert to Dynamic Data"("Array"=w519) -> ("Dynamic Data Type"=w518:dynamicdata)  [unwired: 3 in]
      n335 = call "Convert to Dynamic Data2"("Array"=w511) -> ("Dynamic Data Type"=w517:dynamicdata)  [unwired: 3 in]
      n336 = call "Convert to Dynamic Data3"("Array"=w511) -> ("Dynamic Data Type"=w516:dynamicdata)  [unwired: 3 in]
      n337 = Merge Signals(w517, w516) -> (w509:dynamicdata)
      n338 = Build Array (concatenate)(w512, w510) -> (w513:dbl[])
      n339 = call "Convert to Dynamic Data4"("Array"=w515) -> ("Dynamic Data Type"=w514:dynamicdata)  [unwired: 3 in]
      n340 = global write "G_ALL.vi" "Steering coeff"(w513) -> ()
      n341 = Merge Signals(w518, w514) -> (w508:dynamicdata)
      n342 = call "Build XY Graph"("Y Input"=w509, "X Input"=w508) -> ("XY Graph"=→"XY Graph":cluster{"X":dbl[], "Y":dbl[]}[])  [unwired: 8 in, 1 out]
    }
  }
